vi "programa6.vi"() -> ()   [LabVIEW 2011]
panel:
  out "Aceptado":bool
  out "Edad":dbl
  in  "Experiencia":u16(ring) items=["Experiencia", "No tiene"]
  in  "Tiene Titulo":u16(ring) items=["No tiene", "Tiene"]
  # "Se debe de seleccionar si tiene o no tiene titulo. luego si tiene experiencia y \ngenerar la edad entre 20-70.\nEs contratado si la edad es mayor a 25 y si tiene experiencia o si tiene titulo\ny no tiene experiencia y es mayor a 25."
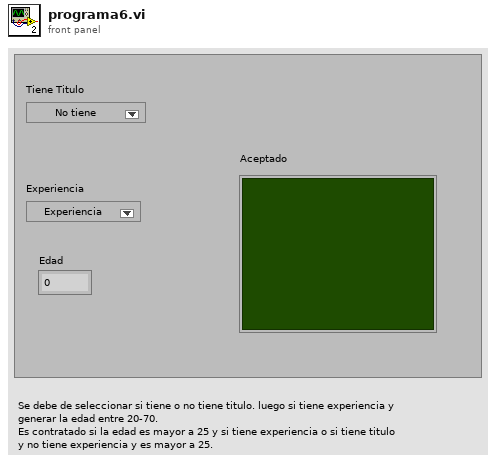
[diagram p1: front panel]
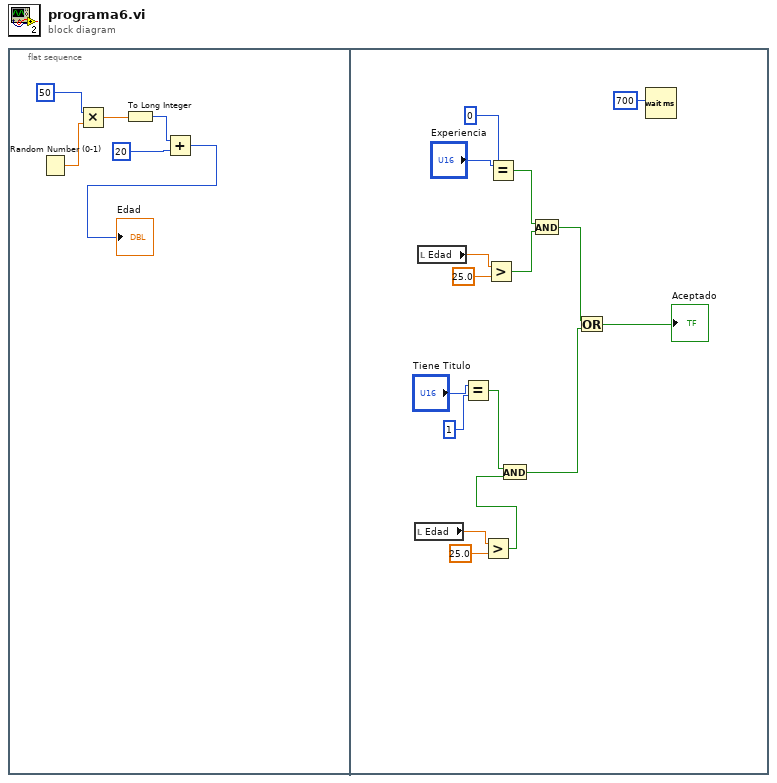
[diagram p0: block diagram]
diagram:
  n1 = flat-sequence {
    frame #0 {
      n2 = Random Number (0-1)() -> (number: 0 to 1=w5:dbl)
      n3 = Multiply(x=50, y=w5) -> (x*y=w4:dbl)
      n4 = To Long Integer(number=w4) -> (32bit integer=w3:i32)
      n5 = Add(x=w3, y=20) -> (x+y=→"Edad":i32)
    }
    frame #1 {
      n6 = local read "Edad"() -> (w15:dbl)
      n7 = local read "Edad"() -> (w22:dbl)
      n8 = Equal?(x="Tiene Titulo", y=u16 1) -> (x = y?=w12:bool)
      n9 = Greater?(x=w15, y=25.0) -> (0:w11:bool)
      n10 = Greater?(x=w22, y=25.0) -> (0:w17:bool)
      n11 = Equal?(x="Experiencia", y=u16 0) -> (x = y?=w18:bool)
      n12 = And(x=w12, y=w11) -> (x .and. y?=w9:bool)
      n13 = And(x=w18, y=w17) -> (x .and. y?=w10:bool)
      n14 = Or(x=w10, y=w9) -> (x .or. y?=→"Aceptado":bool)
      n15 = Wait (ms)(milliseconds to wait=700) -> ()  [unwired: 1 out]
    }
  }
